vi "Get Parameters in Frame.vi"(8 "error in":errorcluster, 11 "word ref":T1 format="%.0x") -> (0 "error out":errorcluster, 1 "parameter definitions":T2[](array[typedef]), 2 "parameter references":T1[](array[typedef]) format="%.0x", 3 "word ref out":T1 format="%.0x")   [LabVIEW 2020, in "Ballard ARINC 429 Scripting.lvlib"]
uses:
  Ballard ARINC 429 Scripting.lvlib
  <vilib>/NI VeriStand/Custom Device API/Custom Device API.lvlib
  <vilib>/NI VeriStand/Custom Device Tools/Custom Device Utility Library/Custom Device Utility Library.lvlib
  <vilib>/NI VeriStand/Custom Device Tools/Custom Device Utility Library/NI VeriStand - Search for Item by GUID.vi
  Constants.vi
  <vilib>/NI VeriStand/Custom Device API/Custom Device Item Ref.ctl
  Encoding and Decoding/Encoding.ctl
  Encoding and Decoding/Encoding and Decoding.lvlib
  Shared/Parameter Definition.ctl
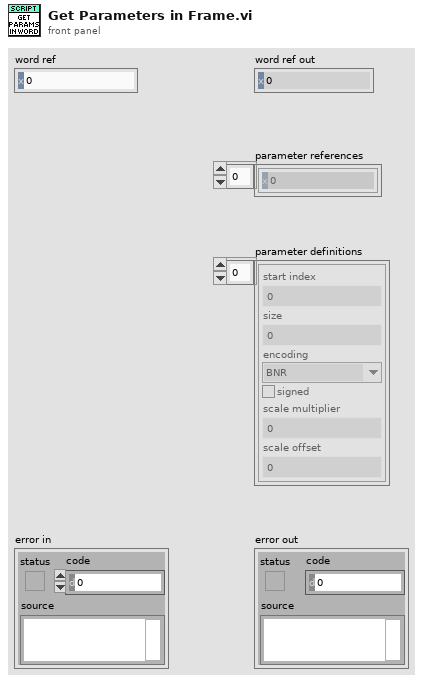
[diagram p1: front panel]
types:
  T1 = typedef "Custom Device API.lvlib/Custom Device Item Ref.ctl" = u64
  T2 = typedef "Parameter Definition.ctl" = cluster{"start index":i32, "size":i32, "encoding":T3, "signed":bool, "scale multiplier":dbl, "scale offset":dbl}
  T3 = typedef "Encoding and Decoding.lvlib/Encoding.ctl" = enum16{"BNR", "BCD", "Discrete"}
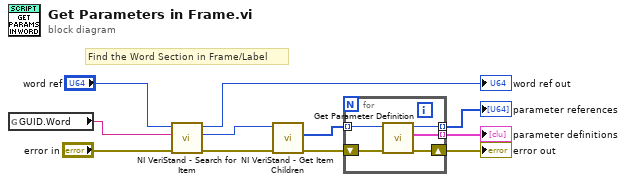
[diagram p0: block diagram]
diagram:
  # "Find the Word Section in Frame/Label"
  n1 = global read "Constants.vi" "GUID.Word"() -> (w1:string)
  n2 = call-poly <vilib>:"NI VeriStand - Search for Item.vi"("error in"="error in", "Item GUID"=w1, "Section Ref in"="word ref") -> ("error out"=w5:errorcluster, "Item Ref"=w4:T1, "Section Ref out"=→"word ref out":T1)  [unwired: 5 in, 1 out]
  n3 = call <vilib>:"NI VeriStand - Get Item Children.vi"("error in (no error)"=w5, "Item Ref in"=w4) -> ("error out"=w11:errorcluster, "Child Refs"=w9:T1[])  [unwired: 6 in, 2 out]
  n4 = for {
    shift-right: [w15] -> w10
    shift-left: w11 -> [w16]
    tunnel: w9 -> [w14] mode=indexing
    tunnel: [w13] -> w8 mode=indexing
    tunnel: [w12] -> w7 mode=indexing
    n5 = call "Get Parameter Definition.vi"("error in"=w16, "parameter ref in"=w14) -> ("error out"=w15:errorcluster, "parameter definition"=w13:T2, "parameter ref out"=w12:T1)  [unwired: 7 in]
  }
  "error out" <- w10
  "parameter definitions" <- w8
  "parameter references" <- w7
